vi "PowerControl.vi"(8 "error in":errorcluster, 10 "Pulses\n(/0.45°)":u16=44, 11 "Direction":bool) -> (0 "error out":errorcluster)   [LabVIEW 2015]
uses:
  <vilib>/DAQmx/write.llb/DAQmx Write (Digital Bool 1Line 1Point).vi
  <vilib>/DAQmx/create/channels.llb/DAQmx Create Channel (DO-Digital Output).vi
  <vilib>/DAQmx/miscellaneous.llb/DAQmx Fill In Error Info.vi
  <vilib>/DAQmx/create/channels.llb/DAQmx Create Channel (CO-Pulse Generation-Frequency).vi
  <vilib>/DAQmx/configure/timing.llb/DAQmx Timing (Implicit).vi
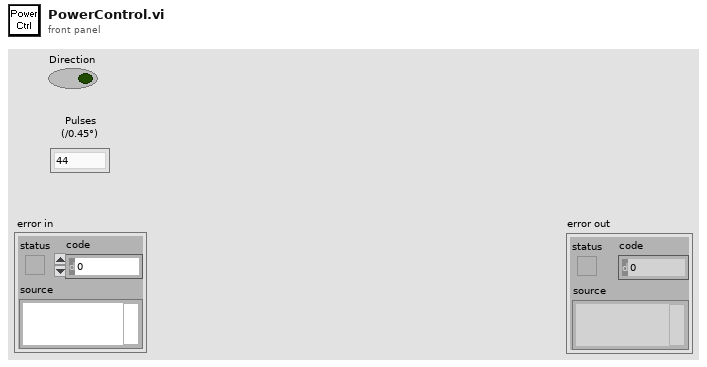
[diagram p1: front panel]
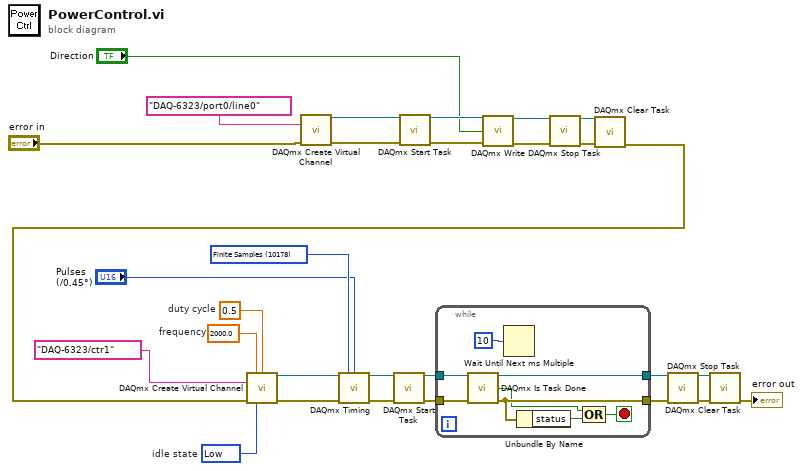
[diagram p0: block diagram]
diagram:
  w14 = 10214 items=["High"=10192, "Low"=10214]  # idle state
  w15 = 0.5  # duty cycle
  w24 = 2000.0  # frequency
  w26 = 10178 items=["Finite Samples"=10178, "Continuous Samples"=10123] ("sample mode")
  n1 = call-poly <vilib>:"DAQmx Create Virtual Channel.vi"("lines"=tag "DAQ-6323/port0/line0", "error in"="error in") -> ("task out"=w12:refnum<k21>, "error out"=w13:errorcluster)  [unwired: 12 in]
  n2 = call <vilib>:"DAQmx Start Task.vi"("task/channels in"=w12, "error in"=w13) -> ("task out"=w11:refnum<k21>, "error out"=w10:errorcluster)  [unwired: 12 in]
  n3 = call-poly <vilib>:"DAQmx Write.vi"("task/channels in"=w11, "data"="Direction", "error in"=w10) -> ("task out"=w7:refnum<k21>, "error out"=w6:errorcluster)  [unwired: 10 in, 1 out]
  n4 = call <vilib>:"DAQmx Stop Task.vi"("task/channels in"=w7, "error in"=w6) -> ("task out"=w9:refnum<k21>, "error out"=w8:errorcluster)  [unwired: 12 in]
  n5 = call <vilib>:"DAQmx Clear Task.vi"("task in"=w9, "error in"=w8) -> ("error out"=w3:errorcluster)  [unwired: 13 in]
  n6 = call-poly <vilib>:"DAQmx Create Virtual Channel.vi"("frequency"=w24, "duty cycle"=w15, "counter"=tag "DAQ-6323/ctr1", "error in"=w3, "idle state"=w14) -> ("task out"=w27:refnum<k21>, "error out"=w29:errorcluster)  [unwired: 9 in]
  n7 = call-poly <vilib>:"DAQmx Timing.vi"("task/channels in"=w27, "sample mode"=w26, "samples per channel"="Pulses\n(/0.45°)", "error in"=w29) -> ("task out"=w23:refnum<k21>, "error out"=w22:errorcluster)  [unwired: 10 in]
  n8 = call <vilib>:"DAQmx Start Task.vi"("task/channels in"=w23, "error in"=w22) -> ("task out"=w21:refnum<k21>, "error out"=w20:errorcluster)  [unwired: 12 in]
  n9 = while {
    tunnel: w21 -> [w37]
    tunnel: w20 -> [w36]
    tunnel: [w33] -> w18
    tunnel: [w34] -> w19
    stop <- w35 stop-if-true
    n10 = call <vilib>:"DAQmx Is Task Done.vi"("task/channels in"=w37, "error in"=w36) -> ("task out"=w34:refnum<k21>, "task done?"=w30:bool, "error out"=w33:errorcluster)  [unwired: 11 in]
    n11 = Wait Until Next ms Multiple(millisecond multiple=u32 10) -> ()  [unwired: 1 out]
    n12 = Unbundle By Name(w33) -> ("status"=w32:bool)
    n13 = Compound Arithmetic op=OR(w30, w32) -> (w35:bool)
  }
  n14 = call <vilib>:"DAQmx Stop Task.vi"("task/channels in"=w19, "error in"=w18) -> ("task out"=w17:refnum<k21>, "error out"=w16:errorcluster)  [unwired: 12 in]
  n15 = call <vilib>:"DAQmx Clear Task.vi"("task in"=w17, "error in"=w16) -> ("error out"=→"error out":errorcluster)  [unwired: 13 in]
